vi "15_TimeDifferences_setup.vi"(5 "click_channel":i32(ring) items=["1 (Standard)"=1, "2 (Standard)"=2, "3 (Standard)"=3, "4 (Standard)"=4, "5 (Standard)"=5, "6 (Standard)"=6, "7 (Standard)"=7, "8 (Standard)"=8, "9 (Standard)"=9, "10 (Standard)"=10, "11 (Standard)"=11, "12 (Standard)"=12, "13 (Standard)"=13, "14 (Standard)"=14, "15 (Standard)"=15, "16 (Standard)"=16, "17 (Standard)"=17, "18 (Standard)"=18], 7 "start_channel":i32(ring) items=["1 (Standard)"=1, "2 (Standard)"=2, "3 (Standard)"=3, "4 (Standard)"=4, "5 (Standard)"=5, "6 (Standard)"=6, "7 (Standard)"=7, "8 (Standard)"=8, "9 (Standard)"=9, "10 (Standard)"=10, "11 (Standard)"=11, "12 (Standard)"=12, "13 (Standard)"=13, "14 (Standard)"=14, "15 (Standard)"=15, "16 (Standard)"=16, "17 (Standard)"=17, "18 (Standard)"=18], 8 "error in (no error)":errorcluster, 11 "TimeTagger ref in":refnum<k24>) -> (0 "error out":errorcluster, 2 "TimeDifferences ref out":refnum<k24>, 3 "TimeTagger ref out":refnum<k24>)   [LabVIEW 2014]
doc: "Set up the TimeDifferences measurement and switch on the internal test signal."
uses:
  SwabianInstruments.TimeTagger
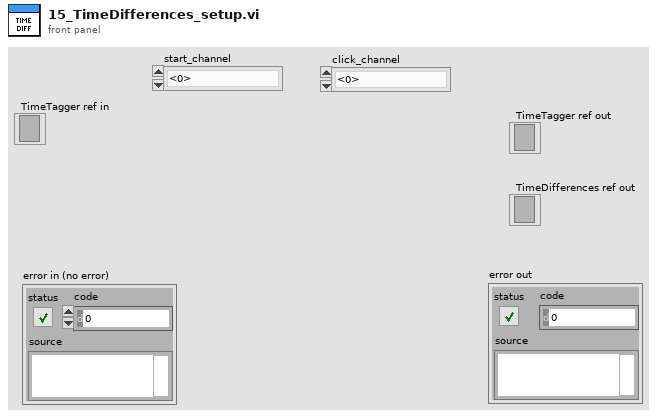
[diagram p1: front panel]
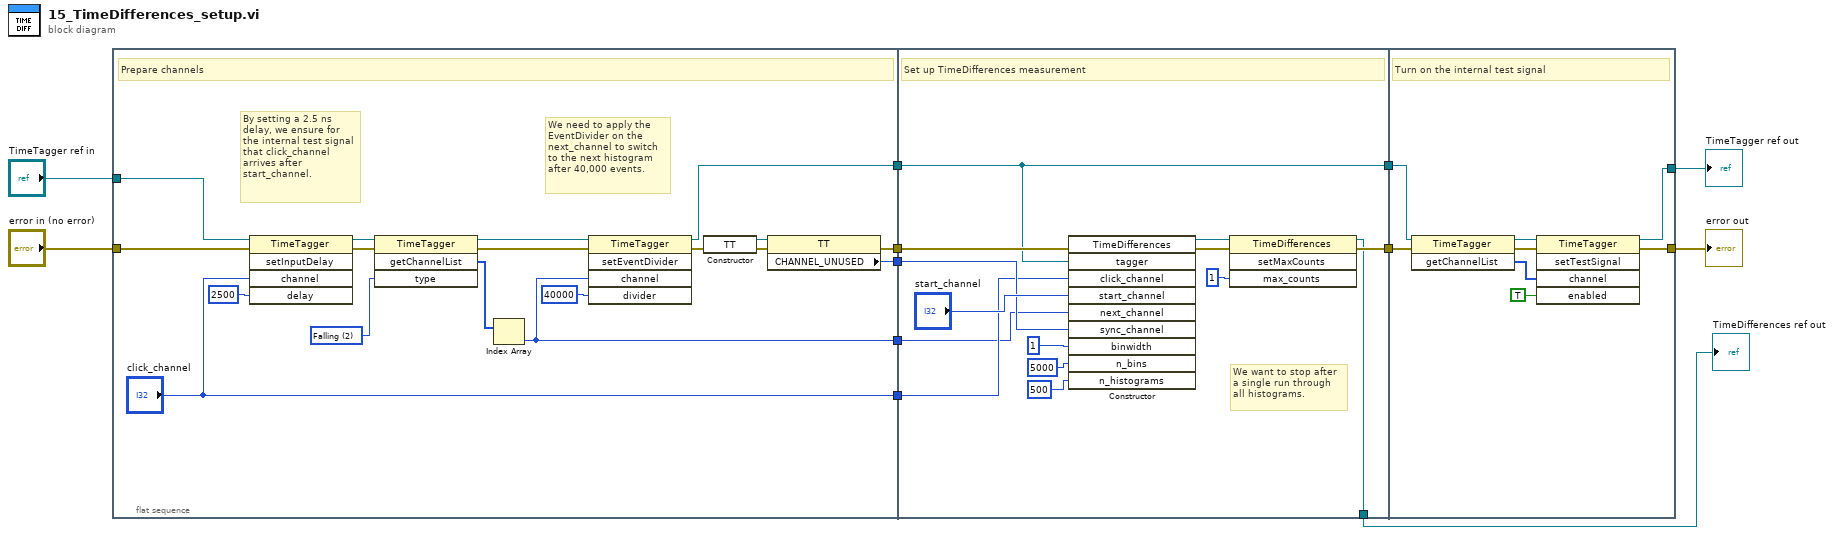
[diagram p0: block diagram]
diagram:
  n1 = flat-sequence {
    tunnel: [w19] -> w12
    tunnel: [w18] -> w11
    tunnel: [w17] -> w10
    tunnel: ["click_channel"] -> w9
    tunnel: [w15] -> w8
    tunnel: "TimeTagger ref in" -> [w14]
    tunnel: "error in (no error)" -> [w13]
    tunnel: w12 -> [w37]
    tunnel: w11 -> [w35]
    tunnel: w10 -> [w34]
    tunnel: w9 -> [w33]
    tunnel: w8 -> [w32]
    tunnel: [w36] -> w7
    tunnel: [w35] -> w6
    tunnel: [w31] -> w1
    tunnel: [w50] -> w5
    tunnel: [w51] -> w4
    tunnel: w7 -> [w48]
    tunnel: w6 -> [w49]
    frame #0 {
      w28 = 2 items=["All"=0, "Rising"=1, "Falling"=2, "HighResAll"=4, "HighResRising"=5, "HighResFalling"=6, "StandardAll"=8, "StandardRising"=9, "StandardFalling"=10] ("type")
      # "We need to apply the\nEventDivider on the\nnext_channel to switch\nto the next histogram\nafter 40,000 events."
      # "By setting a 2.5 ns\ndelay, we ensure for\nthe internal test signal\nthat click_channel\narrives after\nstart_channel."
      # "Prepare channels"
      n2 = invoke class="TimeTagger" method="setInputDelay"(reference=w14, error in=w13, "channel"="click_channel", "delay"=i64 2500) -> (reference out=w24:refnum<k24>, error out=w25:errorcluster)  [unwired: 1 in, 3 out]
      n3 = invoke class="TimeTagger" method="getChannelList"(reference=w24, error in=w25, "type"=w28) -> (reference out=w22:refnum<k24>, error out=w23:errorcluster, "getChannelList"=w27:i32[])  [unwired: 1 in, 1 out]
      n4 = Index Array(array=w27) -> (element=w15:i32)  [unwired: 1 in]
      n5 = invoke class="TimeTagger" method="setEventDivider"(reference=w22, error in=w23, "channel"=w15, "divider"=u32 40000) -> (reference out=w18:refnum<k24>, error out=w21:errorcluster)  [unwired: 1 in, 3 out]
      n6 = constructor class="TT"(error in=w21) -> (reference out=w30:refnum<k24>, error out=w29:errorcluster)  [unwired: 2 in, 1 out]
      n7 = property class="TT"(reference=w30, error in=w29) -> (error out=w19:errorcluster, "CHANNEL_UNUSED"=w17:i32)  [unwired: 1 out]
    }
    frame #1 {
      # "We want to stop after\na single run through\nall histograms."
      # "Set up TimeDifferences measurement"
      n8 = constructor class="TimeDifferences"(error in=w37, "tagger"=w35, "click_channel"=w33, "start_channel"="start_channel", "next_channel"=w32, "sync_channel"=w34, "binwidth"=i64 1, "n_bins"=5000, "n_histograms"=500) -> (reference out=w39:refnum<k24>, error out=w41:errorcluster)  [unwired: 2 in, 9 out]
      n9 = invoke class="TimeDifferences" method="setMaxCounts"(reference=w39, error in=w41, "max_counts"=u64 1) -> (reference out=w31:refnum<k24>, error out=w36:errorcluster)  [unwired: 1 in, 2 out]
    }
    frame #2 {
      # "Turn on the internal test signal"
      n10 = invoke class="TimeTagger" method="getChannelList"(reference=w49, error in=w48) -> (reference out=w47:refnum<k24>, error out=w46:errorcluster, "getChannelList"=w45:i32[])  [unwired: 1 in]
      n11 = invoke class="TimeTagger" method="setTestSignal"(reference=w47, error in=w46, "channel"=w45, "enabled"=TRUE) -> (reference out=w51:refnum<k24>, error out=w50:errorcluster)  [unwired: 1 in, 3 out]
    }
  }
  "error out" <- w5
  "TimeTagger ref out" <- w4
  "TimeDifferences ref out" <- w1
